vi "关闭数控.vi"(8 "error in (no error)":errorcluster, 11 "ADODB._Connection In":refnum<k7>) -> (0 "error out":errorcluster)   [LabVIEW 2013]
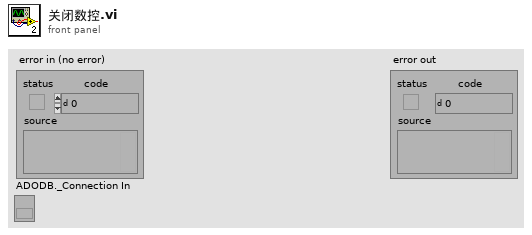
[diagram p1: front panel]
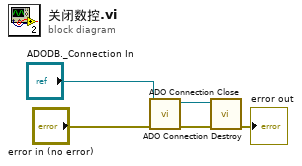
[diagram p0: block diagram]
diagram:
  n1 = call "ADO Connection Close.vi"("error in (no error)"="error in (no error)", "ADODB._Connection In"="ADODB._Connection In") -> ("error out"=w5:errorcluster, "ADODB._Connection Out"=w4:refnum<k7>)  [unwired: 8 in]
  n2 = call "ADO Connection Destroy.vi"("error in (no error)"=w5, "ADODB._Connection In"=w4) -> ("error out"=→"error out":errorcluster)  [unwired: 9 in]
